vi "command_move_relative.vi"(8 "error in (no error)":errorcluster, 10 "target  position":refnum<class "SpaceVector.lvclass">, 11 "StageMH110930Scientifica in":refnum<class "StageMMS2015ASIfromScientifica.lvclass">) -> (0 "error out":errorcluster, 3 "StageMH110930Scientifica out":refnum<class "StageMMS2015ASIfromScientifica.lvclass">)   [LabVIEW 2010, in "StageMMS2015ASIfromScientifica.lvclass"]
uses:
  StageMMS2015ASIfromScientifica.lvclass
  common/classes/SpaceVector/SpaceVector/SpaceVector.lvclass
  common/classes/ErrorController/ErrorController/class_data.vi
  common/classes/ErrorController/ErrorController/ErrorController.lvclass
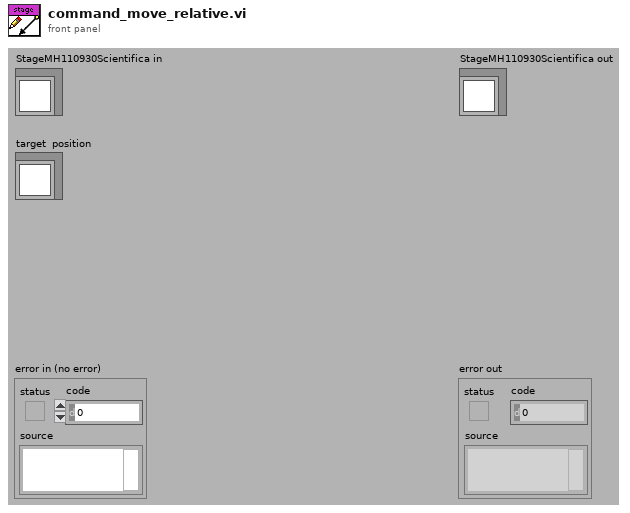
[diagram p1: front panel]
types:
  T1 = typedef "SpaceVector.lvclass/space_vector_array.ctl" = dbl[unit][]
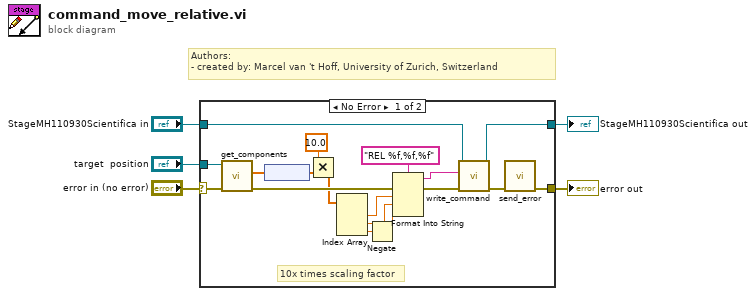
[diagram p0: block diagram]
diagram:
  # "Authors: \n- created by: Marcel van 't Hoff, University of Zurich, Switzerland"
  n1 = case shown="No Error" "error in (no error)" {
    selector: "error in (no error)" -> [w22 w25]
    tunnel: [w11 w25] -> w4
    tunnel: [w12 w24] -> w2
    tunnel: "StageMH110930Scientifica in" -> [w13 w24]
    tunnel: "target  position" -> [w23 _]
    frame No Error {
      # "10x times scaling factor"
      n2 = call "get_components.vi"("error in (no error)"=w22, "SpaceVector in"=w23) -> ("error out"=w15:errorcluster, "x/y/z"=w21:T1)  [unwired: 8 out]
      n3 = node(w21) -> (w10:dbl[])
      n4 = Multiply(x=10.0, y=w10) -> (x*y=w8:dbl[])
      n5 = Index Array(array=w8) -> (element #1=w20:dbl, element #2=w19:dbl, element #3=w18:dbl)  [unwired: 3 in]
      n6 = Negate(x=w18) -> (-x=w6:dbl)
      n7 = Format Into String(format string="REL %f,%f,%f", error in=w15, w20, w19, w6) -> (resulting string=w16:string, error out=w14:errorcluster)  [unwired: 1 in]
      n8 = call-dynamic "write_command.vi"("error in (no error)"=w14, "string to write"=w16, "StageMH110930Scientifica in"=w13) -> ("error out"=w9:errorcluster, "StageMH110930Scientifica out"=w12:refnum<class "StageMMS2015ASIfromScientifica.lvclass">)  [unwired: 5 in, 2 out]
      n9 = call "send_error.vi"("error in (no error)"=w9) -> ("error out"=w11:errorcluster)  [unwired: 10 in]
    }
    frame Error {
    }
  }
  "error out" <- w4
  "StageMH110930Scientifica out" <- w2
